vi "time_keeping.vi"(11 "Reset":bool) -> (3 "Time(secs)":dbl)   [LabVIEW 2019]
panel:
  in  "stop":bool
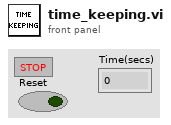
[diagram p1: front panel]
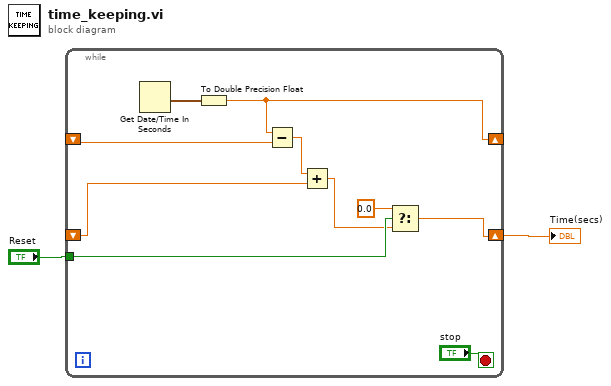
[diagram p0: block diagram]
diagram:
  n1 = while {
    shift-right: [w10] -> _
    shift-left: _ -> [w9]
    shift-right: [w3] -> w2
    shift-left: _ -> [w7]
    tunnel: "Reset" -> [w5]
    stop <- "stop" stop-if-true
    n2 = Get Date/Time In Seconds() -> (seconds since 1Jan1904=w11:timestamp)
    n3 = To Double Precision Float(number=w11) -> (double precision float=w10:dbl)
    n4 = Subtract(x=w10, y=w9) -> (x-y=w8:dbl)
    n5 = Add(x=w8, y=w7) -> (x+y=w4:dbl)
    n6 = Select(t=0.0, s=w5, f=w4) -> (s? t:f=w3:dbl)
  }
  "Time(secs)" <- w2
